vi "EXERON JSON.vi"(5 "Boolean":bool, 6 "Baterias":refnum<class "JSON Object.lvclass">=refnum, 7 "JSON Object in":refnum<class "JSON Object.lvclass">=refnum, 8 "error in":errorcluster, 9 "CARGA":refnum<class "JSON Array.lvclass">=refnum, 10 "FV":refnum<class "JSON Object.lvclass">=refnum, 11 "Alarmas":refnum<class "JSON Array.lvclass">=refnum) -> (0 "error out":errorcluster, 3 "JSON Object out":refnum<class "JSON Object.lvclass">)   [LabVIEW 2015]
uses:
  <vilib>/addons/JSON API/JSON Object/Set Object Item by name.vi
  <vilib>/addons/JSON API/JSON Object/JSON Object.lvclass
  <vilib>/addons/JSON API/JSON Array/JSON Array.lvclass
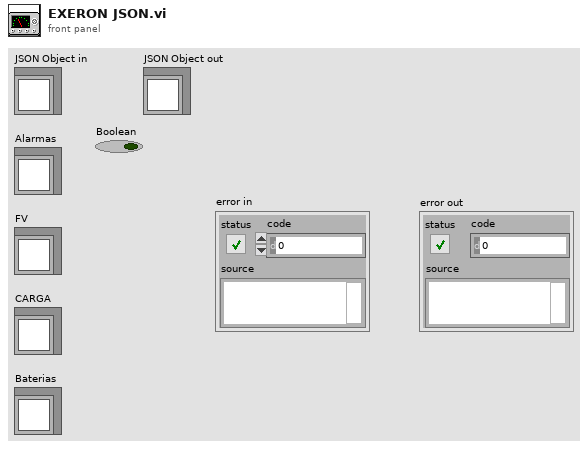
[diagram p1: front panel]
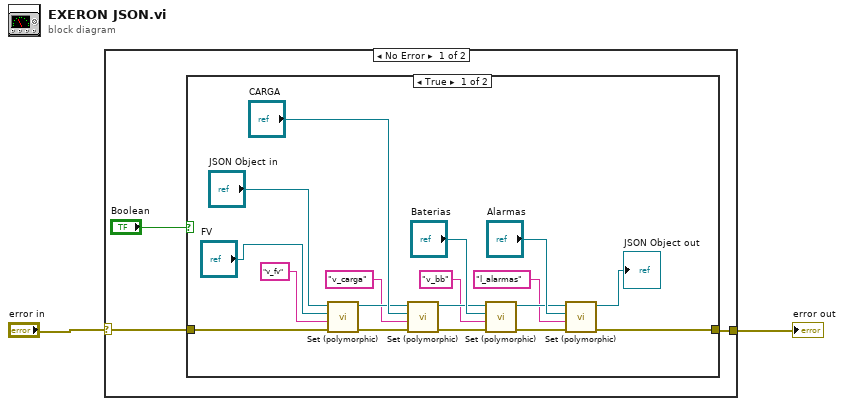
[diagram p0: block diagram]
diagram:
  n1 = case shown="No Error" "error in" {
    selector: "error in" -> [w3 w25]
    tunnel: [w5 w25] -> w2
    frame No Error {
      n2 = case shown="True" "Boolean" {
        tunnel: [w17 w24] -> w5
        tunnel: w3 -> [w6 w24]
        frame True {
          n3 = call-poly <vilib>:"Set (polymorphic).vi"("error in (no error)"=w6, "name"="v_fv", "Value"="FV", "JSON Object in"="JSON Object in") -> ("error out"=w13:errorcluster, "JSON Object out"=w16:refnum<class "JSON Object.lvclass">)  [unwired: 5 in, 1 out]
          n4 = call-poly <vilib>:"Set (polymorphic).vi"("error in (no error)"=w13, "name"="v_carga", "Value"="CARGA", "JSON Object in"=w16) -> ("error out"=w12:errorcluster, "JSON Object out"=w15:refnum<class "JSON Object.lvclass">)  [unwired: 5 in, 1 out]
          n5 = call-poly <vilib>:"Set (polymorphic).vi"("error in (no error)"=w12, "name"="v_bb", "Value"="Baterias", "JSON Object in"=w15) -> ("error out"=w11:errorcluster, "JSON Object out"=w14:refnum<class "JSON Object.lvclass">)  [unwired: 5 in, 1 out]
          n6 = call-poly <vilib>:"Set (polymorphic).vi"("error in (no error)"=w11, "name"="l_alarmas", "Value"="Alarmas", "JSON Object in"=w14) -> ("error out"=w17:errorcluster, "JSON Object out"=→"JSON Object out":refnum<class "JSON Object.lvclass">)  [unwired: 5 in, 1 out]
        }
        frame False {
        }
      }
    }
    frame Error {
    }
  }
  "error out" <- w2
